vi "Draw Assert Data.vi"(8 "error in (no error)":errorcluster, 10 "Assert Array":T1[](array[typedef]), 11 "UserInterface in":refnum<class "UserInterface.lvclass">) -> (0 "error out":errorcluster)   [LabVIEW 2016, in "UserInterface.lvlib" / "UserInterface.lvclass"]
uses:
  UserInterface.lvclass
  AssertEngine/Log Assert/Assert Data.ctl
  UserInterface.lvclass/UserInterface.ctl
  AssertEngine/AssertEngine.lvlib
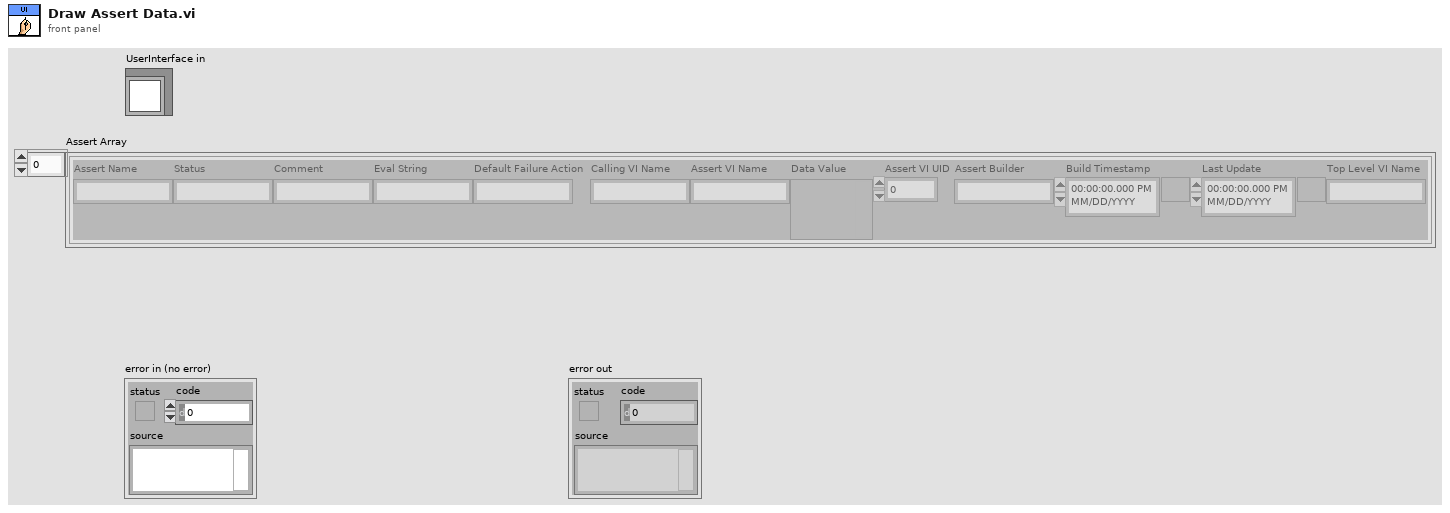
[diagram p1: front panel]
types:
  T1 = typedef "AssertEngine.lvlib/Assert Data.ctl" = cluster{"Assert Name":string, "Status":string, "Comment":string, "Eval String":string, "Default Failure Action":string, "Calling VI Name":string, "Assert VI Name":string, "Data Value":variant, "Assert VI UID":i32, "Assert Builder":string, "Build Timestamp":timestamp, "Last Update":timestamp, "Top Level VI Name":string}
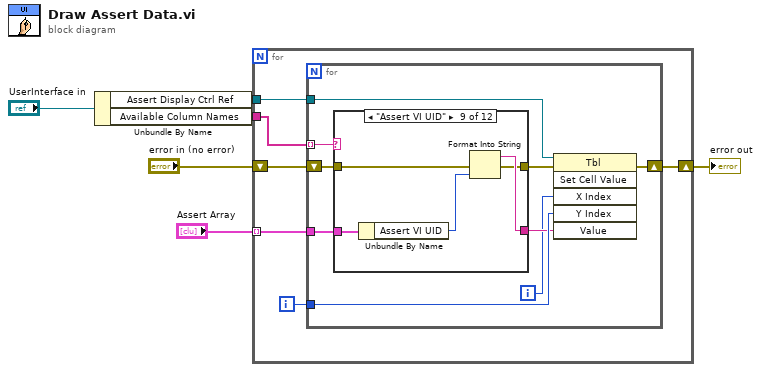
[diagram p0: block diagram]
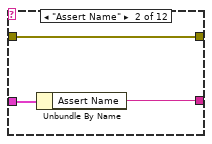
[diagram p3: hidden frame]
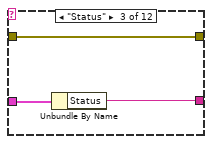
[diagram p4: hidden frame]
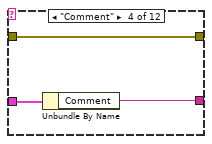
[diagram p5: hidden frame]
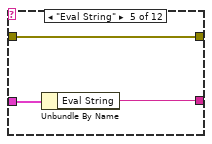
[diagram p6: hidden frame]
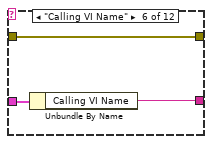
[diagram p7: hidden frame]
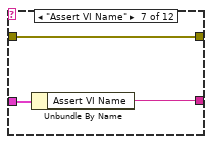
[diagram p8: hidden frame]
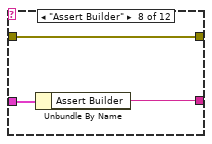
[diagram p9: hidden frame]
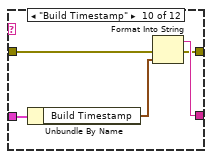
[diagram p10: hidden frame]
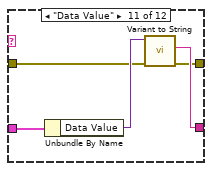
[diagram p11: hidden frame]
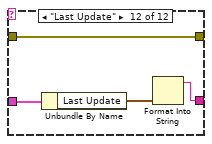
[diagram p12: hidden frame]
diagram:
  n1 = Unbundle By Name("UserInterface in") -> ("Assert Display Ctrl Ref"=w3:refnum<vi>, "Available Column Names"=w4:string[])
  n2 = for {
    tunnel: "Assert Array" -> [w12] mode=indexing
    tunnel: w4 -> [w7]
    tunnel: w3 -> [w10]
    shift-right: [w8] -> w1
    shift-left: "error in (no error)" -> [w9]
    i -> [w11]
    n3 = for {
      tunnel: w12 -> [w21]
      tunnel: w11 -> [w20]
      tunnel: w10 -> [w19]
      shift-right: [w18] -> w8
      shift-left: w9 -> [w14]
      tunnel: w7 -> [w17] mode=indexing
      i -> [w15]
      n4 = case shown="\"Assert VI UID\"" w17 {
        tunnel: w21 -> [_ w25 w28 w31 w34 w37 w40 w43 w48 w53 w58 w62]
        tunnel: [_ w24 w27 w30 w33 w36 w39 w42 w46 w51 w56 w60] -> w16
        tunnel: w14 -> [w22 w23 w26 w29 w32 w35 w38 w41 w45 w50 w55 w59]
        tunnel: [w22 w23 w26 w29 w32 w35 w38 w41 w44 w49 w54 w59] -> w13
        frame Default {
        }
        frame "Assert Name" {
          n5 = Unbundle By Name(w25) -> ("Assert Name"=w24:string)
        }
        frame "Status" {
          n6 = Unbundle By Name(w28) -> ("Status"=w27:string)
        }
        frame "Comment" {
          n7 = Unbundle By Name(w31) -> ("Comment"=w30:string)
        }
        frame "Eval String" {
          n8 = Unbundle By Name(w34) -> ("Eval String"=w33:string)
        }
        frame "Calling VI Name" {
          n9 = Unbundle By Name(w37) -> ("Calling VI Name"=w36:string)
        }
        frame "Assert VI Name" {
          n10 = Unbundle By Name(w40) -> ("Assert VI Name"=w39:string)
        }
        frame "Assert Builder" {
          n11 = Unbundle By Name(w43) -> ("Assert Builder"=w42:string)
        }
        frame "Assert VI UID" {
          n12 = Unbundle By Name(w48) -> ("Assert VI UID"=w47:i32)
          n13 = Format Into String(error in=w45, w47) -> (resulting string=w46:string, error out=w44:errorcluster)  [unwired: 2 in]
        }
        frame "Build Timestamp" {
          n14 = Unbundle By Name(w53) -> ("Build Timestamp"=w52:timestamp)
          n15 = Format Into String(error in=w50, w52) -> (resulting string=w51:string, error out=w49:errorcluster)  [unwired: 2 in]
        }
        frame "Data Value" {
          n16 = Unbundle By Name(w58) -> ("Data Value"=w57:variant)
          n17 = call "Variant to String.vi"("error in (no error)"=w55, "Data Value"=w57) -> ("error out"=w54:errorcluster, "Data Value String"=w56:string)  [unwired: 8 in]
        }
        frame "Last Update" {
          n18 = Unbundle By Name(w62) -> ("Last Update"=w61:timestamp)
          n19 = Format Into String(w61) -> (resulting string=w60:string)  [unwired: 3 in, 1 out]
        }
      }
      n20 = invoke class="Tbl" method="Set Cell Value"(reference=w19, error in=w13, "X Index"=w15, "Y Index"=w20, "Value"=w16) -> (error out=w18:errorcluster)  [unwired: 1 in, 5 out]
    }
  }
  "error out" <- w1
